vi "Motors Move Relative Bk.vi"(2 "Direction":string, 5 "Button":refnum<vi>, 7 "Jog-Mode":bool, 8 "error in":errorcluster, 9 "Distance (mm)":dbl, 10 "Axis":i32, 11 "VISA in":refnum<visa-resource-name>) -> (0 "error out":errorcluster, 3 "VISA out":refnum<visa-resource-name>, 4 "Error Message(s)":string, 6 "Error":bool)   [LabVIEW 2010]
panel:
  out "read buffer loop":string
  out "read buffer 1":string
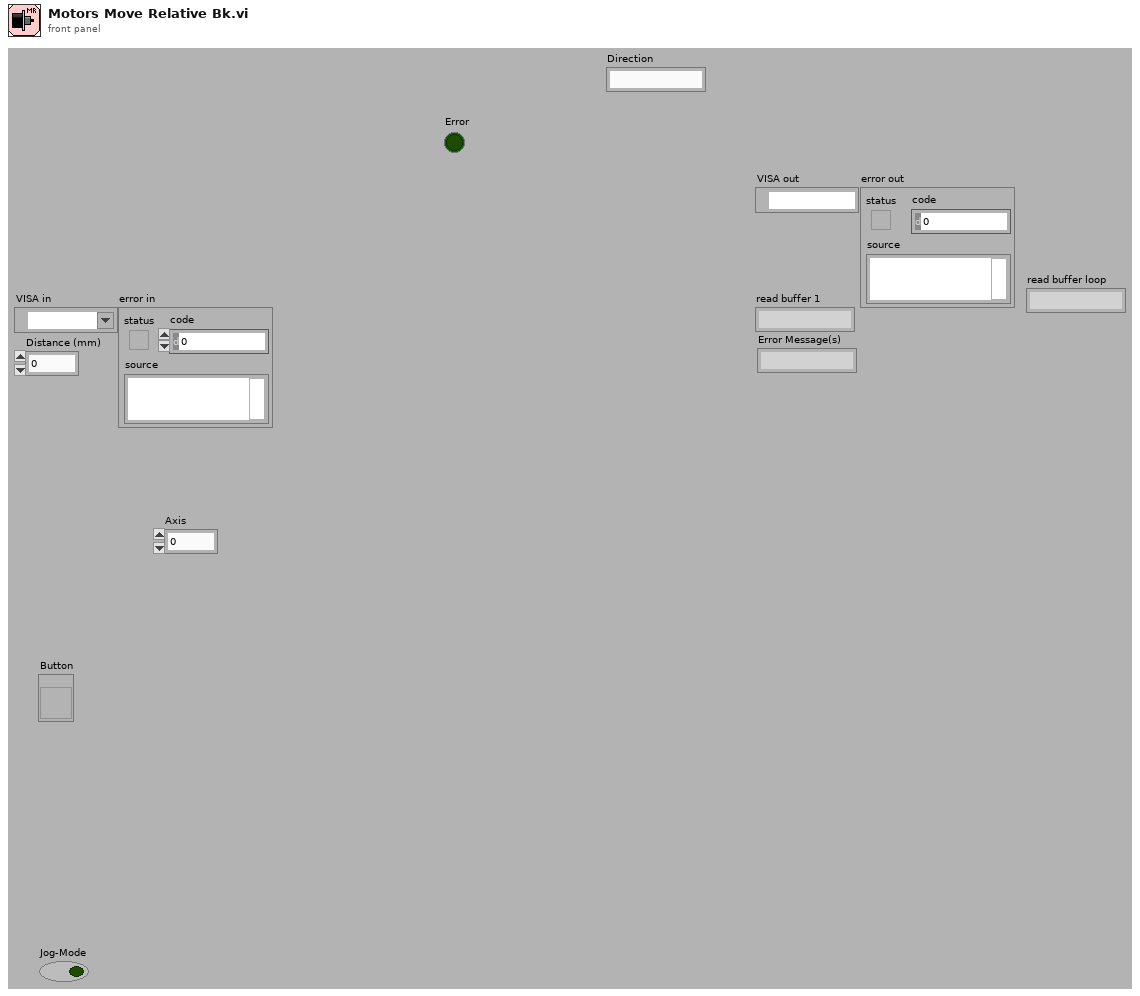
[diagram p1: front panel]
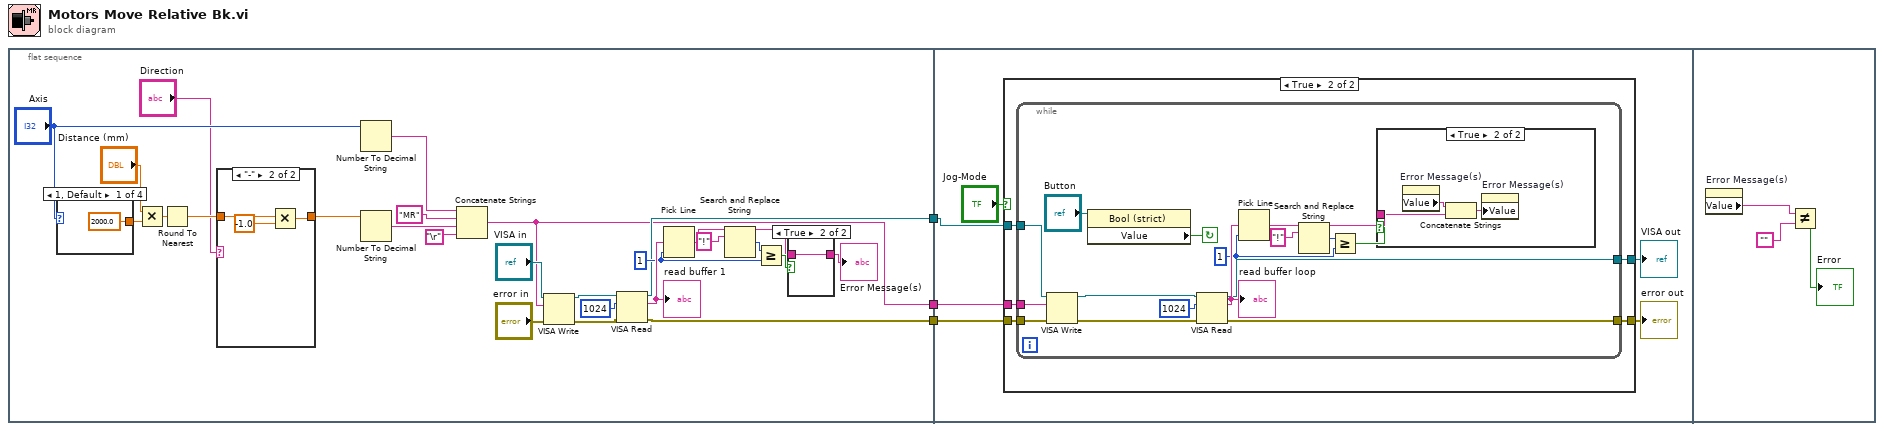
[diagram p0: block diagram]
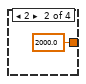
[diagram p4: hidden frame]
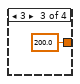
[diagram p5: hidden frame]
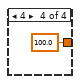
[diagram p6: hidden frame]
diagram:
  n1 = flat-sequence {
    tunnel: [w9] -> w3
    tunnel: [w8] -> w2
    tunnel: [w7] -> w1
    tunnel: w3 -> [w42]
    tunnel: w2 -> [w41]
    tunnel: w1 -> [w40]
    frame #0 {
      w13 = 1 ("line index")
      n2 = case shown="1, Default" "Axis" {
        tunnel: [2000.0 ("y") 2000.0 ("y") 200.0 ("y") 100.0 ("y")] -> w21
        frame 1, Default {
        }
        frame 2 {
        }
        frame 3 {
        }
        frame 4 {
        }
      }
      n3 = Multiply(x="Distance (mm)", y=w21) -> (x*y=w19:dbl)
      n4 = Round To Nearest(number=w19) -> (nearest integer value=w6:dbl)
      n5 = case shown="\"-\"" "Direction" {
        tunnel: w6 -> [w31 w33]
        tunnel: [w31 w34] -> w5
        frame "+", Default {
        }
        frame "-" {
          n6 = Multiply(x=w33, y=-1.0) -> (x*y=w34:dbl)
        }
      }
      n7 = Number To Decimal String(number="Axis") -> (decimal integer string=w28:string)  [unwired: 1 in]
      n8 = Number To Decimal String(number=w5) -> (decimal integer string=w18:string)  [unwired: 1 in]
      n9 = Concatenate Strings(w28, "MR" ("string"), w18, "\r") -> (w7:string)
      n10 = VISA Write(VISA resource name="VISA in", write buffer=w7, error in (no error)="error in") -> (VISA resource name out=w26:refnum<visa-resource-name>, error out=w25:errorcluster)  [unwired: 1 out]
      n11 = VISA Read(VISA resource name=w26, byte count=u32 1024, error in (no error)=w25) -> (VISA resource name out=w9:refnum<visa-resource-name>, read buffer=w16:string, error out=w8:errorcluster)  [unwired: 1 out]
      "read buffer 1" <- w16
      n12 = Pick Line(multi-line string=w16, line index=w13) -> (output string=w17:string)  [unwired: 1 in]
      n13 = Search and Replace String(input string=w17, search string="!" ("search string/char (-)")) -> (result string=w11:string, number of replacements=w14:i32)  [unwired: 6 in, 2 out]
      n14 = Greater Or Equal?(x=w14, y=w13) -> (x >= y?=w12:bool)
      n15 = case shown="True" w12 {
        tunnel: w11 -> [_ w35]
        tunnel: [_ w35] -> w10
        frame False {
        }
        frame True {
        }
      }
      "Error Message(s)" <- w10
    }
    frame #1 {
      n16 = case shown="True" "Jog-Mode" {
        tunnel: w42 -> [w47 w52]
        tunnel: w41 -> [w46 w51]
        tunnel: w40 -> [_ w50]
        tunnel: [w47 w49] -> w44
        tunnel: [w46 w48] -> w45
        frame False {
        }
        frame True {
          n17 = while {
            tunnel: w52 -> [w64]
            tunnel: w51 -> [w63]
            tunnel: w50 -> [w62]
            tunnel: [w54] -> w49
            tunnel: [w53] -> w48
            stop <- w68 continue-if-true
            w58 = 1 ("line index")
            n18 = VISA Write(VISA resource name=w64, write buffer=w62, error in (no error)=w63) -> (VISA resource name out=w65:refnum<visa-resource-name>, error out=w66:errorcluster)  [unwired: 1 out]
            n19 = property class="Bool (strict)"(reference="Button") -> ("Value"=w68:bool)  [unwired: 1 in, 2 out]
            n20 = VISA Read(VISA resource name=w65, byte count=u32 1024, error in (no error)=w66) -> (VISA resource name out=w54:refnum<visa-resource-name>, read buffer=w61:string, error out=w53:errorcluster)  [unwired: 1 out]
            "read buffer loop" <- w61
            n21 = Pick Line(multi-line string=w61, line index=w58) -> (output string=w60:string)  [unwired: 1 in]
            n22 = Search and Replace String(input string=w60, search string="!") -> (result string=w56:string, number of replacements=w59:i32)  [unwired: 6 in, 2 out]
            n23 = Greater Or Equal?(x=w59, y=w58) -> (x >= y?=w57:bool)
            n24 = case shown="True" w57 {
              tunnel: w56 -> [_ w72]
              frame False {
              }
              frame True {
                n25 = property on="Error Message(s)" class="Str"() -> ("Value"=w71:string)  [unwired: 2 in, 2 out]
                n26 = Concatenate Strings(w71, w72) -> (w70:string)
                n27 = property on="Error Message(s)" class="Str"("Value"=w70) -> ()  [unwired: 2 in, 2 out]
              }
            }
          }
        }
      }
      "VISA out" <- w44
      "error out" <- w45
    }
    frame #2 {
      n28 = property on="Error Message(s)" class="Str"() -> ("Value"=w75:string)  [unwired: 2 in, 2 out]
      n29 = Not Equal?(x=w75, y="") -> (x != y?=→"Error":bool)
    }
  }
